vi "to string.vi"(8 "error in":errorcluster, 11 "TDMS datalogger configuration in":refnum<class "TDMS datalogger configuration.lvclass">) -> (0 "error out":errorcluster, 1 "data":string, 2 "version":string, 3 "TDMS datalogger configuration out":refnum<class "TDMS datalogger configuration.lvclass">)   [LabVIEW 2013, in "TDMS datalogger configuration.lvclass"]
doc: "Provides an interface for saving a module configuration to a file or other serialized data source. It is recommended that all children of this class store data in two sets--data required for its own initialization, and any data required for parent initialization--and that each implementation uses the <b>Call Parent Method</b> primitive to serialize parent information."
uses:
  TDMS datalogger configuration.lvclass
  <vilib>/NI/Tag Bus Module Framework/module configuration/TBM module configuration.lvclass
  TDMS datalogger configuration.lvclass/TDMS datalogger configuration.ctl
  <vilib>/NI/Configuration Framework/serializable configuration/NISE_CEF_serializable configuration.lvclass
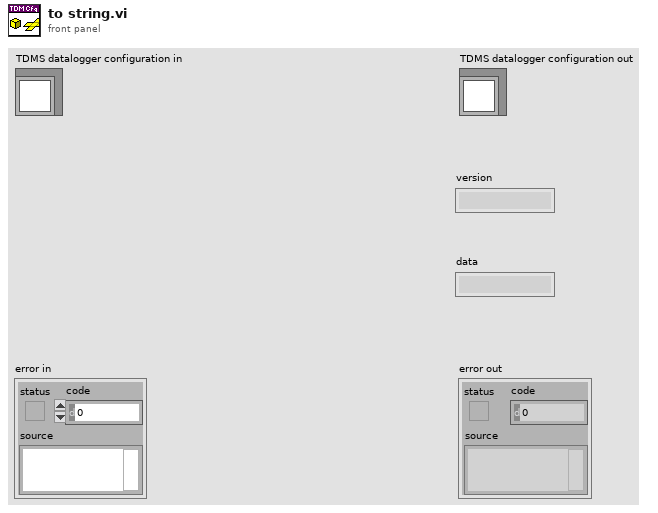
[diagram p1: front panel]
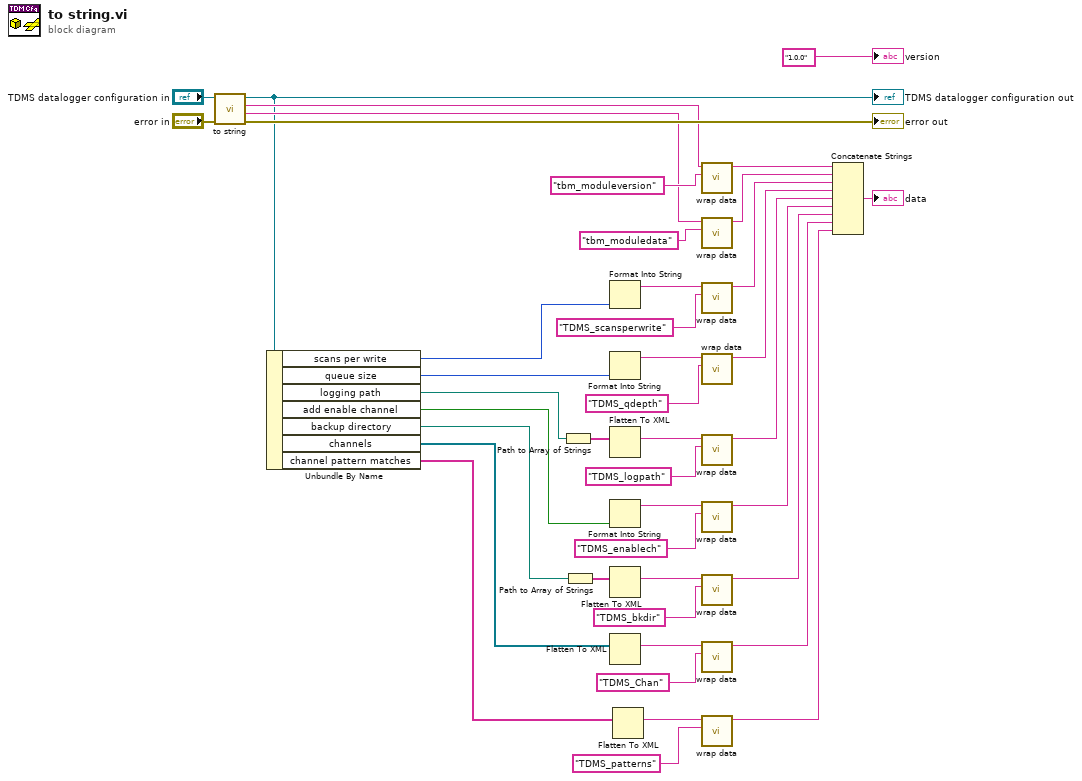
[diagram p0: block diagram]
diagram:
  n1 = call-parent "to string.vi"("error in"="error in", "module configuration in"="TDMS datalogger configuration in") -> ("error out"=→"error out":errorcluster, "data"=w36:string, "version"=w37:string, "module configuration out"=w32:refnum<class "TDMS datalogger configuration.lvclass">)  [unwired: 6 in]
  "TDMS datalogger configuration out" <- w32
  n2 = Unbundle By Name(w32) -> ("scans per write"=w24:i32, "queue size"=w25:i32, "logging path"=w28:path, "add enable channel"=w26:bool, "backup directory"=w30:path, "channels"=w31:refnum<class "TBM channel.lvclass">[], "channel pattern matches"=w5:string[])
  n3 = Path to Array of Strings(0:w28) -> (2:w27:string[])  [unwired: 1 out]
  n4 = Path to Array of Strings(0:w30) -> (2:w29:string[])  [unwired: 1 out]
  n5 = Format Into String(w24) -> (resulting string=w23:string)  [unwired: 3 in, 1 out]
  n6 = Format Into String(w25) -> (resulting string=w21:string)  [unwired: 3 in, 1 out]
  n7 = Flatten To XML(anything=w27) -> (xml string=w19:string)
  n8 = Format Into String(w26) -> (resulting string=w18:string)  [unwired: 3 in, 1 out]
  n9 = Flatten To XML(anything=w29) -> (xml string=w17:string)
  n10 = Flatten To XML(anything=w31) -> (xml string=w16:string)
  n11 = Flatten To XML(anything=w5) -> (xml string=w4:string)
  n12 = call <vilib>:"wrap data.vi"("identifier"="tbm_moduleversion" ("additional identifier"), "data to wrap"=w37) -> ("wrapped data"=w35:string)  [unwired: 9 in]
  n13 = call <vilib>:"wrap data.vi"("identifier"="tbm_moduledata" ("additional identifier"), "data to wrap"=w36) -> ("wrapped data"=w33:string)  [unwired: 9 in]
  n14 = call <vilib>:"wrap data.vi"("identifier"="TDMS_scansperwrite" ("additional identifier"), "data to wrap"=w23) -> ("wrapped data"=w22:string)  [unwired: 9 in]
  n15 = call <vilib>:"wrap data.vi"("identifier"="TDMS_qdepth" ("additional identifier"), "data to wrap"=w21) -> ("wrapped data"=w20:string)  [unwired: 9 in]
  n16 = call <vilib>:"wrap data.vi"("identifier"="TDMS_logpath" ("additional identifier"), "data to wrap"=w19) -> ("wrapped data"=w15:string)  [unwired: 9 in]
  n17 = call <vilib>:"wrap data.vi"("identifier"="TDMS_enablech" ("additional identifier"), "data to wrap"=w18) -> ("wrapped data"=w14:string)  [unwired: 9 in]
  n18 = call <vilib>:"wrap data.vi"("identifier"="TDMS_bkdir" ("additional identifier"), "data to wrap"=w17) -> ("wrapped data"=w13:string)  [unwired: 9 in]
  n19 = call <vilib>:"wrap data.vi"("identifier"="TDMS_Chan" ("additional identifier"), "data to wrap"=w16) -> ("wrapped data"=w12:string)  [unwired: 9 in]
  n20 = call <vilib>:"wrap data.vi"("identifier"="TDMS_patterns", "data to wrap"=w4) -> ("wrapped data"=w2:string)  [unwired: 9 in]
  n21 = Concatenate Strings(w35, w33, w22, w20, w15, w14, w13, w12, w2) -> (→"data":string)
  "version" <- "1.0.0" ("current version")
